vi "Get Boundary of Array.vi"(11 "Array":dbl[](array[numeric])=[0.0, 0.0, 1.0, 2.0, 5.0, 0.0, 0.0, 0.0]) -> (2 "Up":i32, 3 "Down":i32)   [LabVIEW 2024]
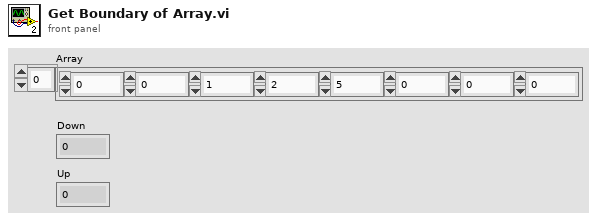
[diagram p1: front panel]
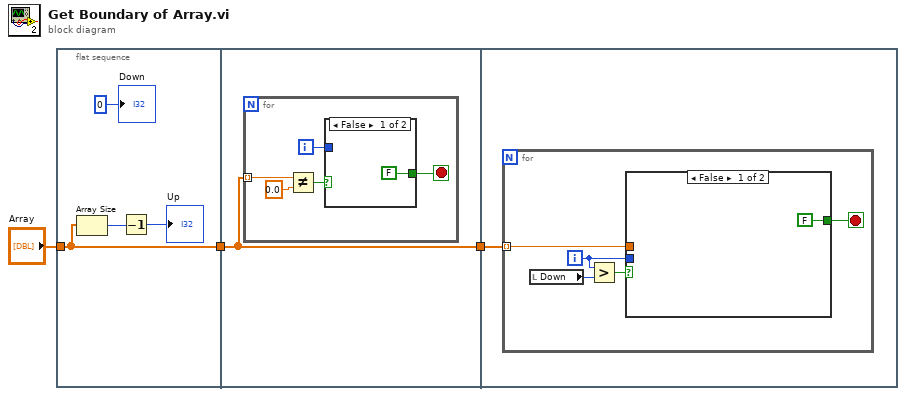
[diagram p0: block diagram]
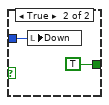
[diagram p2: hidden frame]
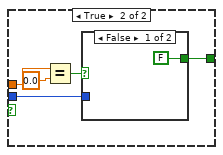
[diagram p3: hidden frame]
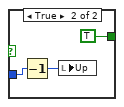
[diagram p4: hidden frame]
diagram:
  n1 = flat-sequence {
    tunnel: "Array" -> [w5]
    tunnel: [w5] -> w2
    tunnel: w2 -> [w8]
    tunnel: [w8] -> w1
    tunnel: w1 -> [w17]
    frame #0 {
      n2 = Array Size(array=w5) -> (size(s)=w7:i32)
      n3 = Decrement(x=w7) -> (x-1=→"Up":i32)
      "Down" <- 0 ("Down")
    }
    frame #1 {
      n4 = for {
        tunnel: w8 -> [w13] mode=indexing
        i -> [w10]
        stop <- w9 stop-if-true
        n5 = Not Equal?(x=w13, y=0.0) -> (x != y?=w11:bool)
        n6 = case shown="False" w11 {
          tunnel: w10 -> [_ w16]
          tunnel: [FALSE TRUE] -> w9
          frame False {
          }
          frame True {
            n7 = local write "Down"(w16) -> ()
          }
        }
      }
    }
    frame #2 {
      n8 = for {
        tunnel: w17 -> [w20] mode=indexing
        i -> [w19]
        stop <- w18 stop-if-true
        n9 = local read "Down"() -> (w22:i32)
        n10 = Greater?(x=w19, y=w22) -> (0:w21:bool)
        n11 = case shown="False" w21 {
          tunnel: w20 -> [_ w28]
          tunnel: w19 -> [_ w25]
          tunnel: [FALSE w24] -> w18
          frame False {
          }
          frame True {
            n12 = Equal?(x=w28, y=0.0) -> (x = y?=w26:bool)
            n13 = case shown="False" w26 {
              tunnel: w25 -> [_ w32]
              tunnel: [FALSE TRUE] -> w24
              frame False {
              }
              frame True {
                n14 = Decrement(x=w32) -> (x-1=w31:i32)
                n15 = local write "Up"(w31) -> ()
              }
            }
          }
        }
      }
    }
  }
